vi "Post-Install Custom Action.vi"(10 "Variant":variant) -> (0 "error out":errorcluster)   [LabVIEW 2021]
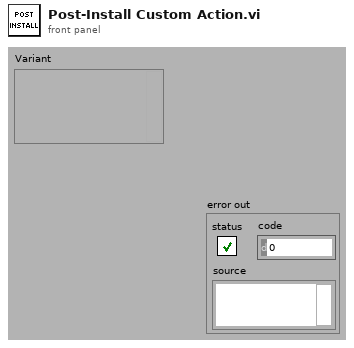
[diagram p1: front panel]
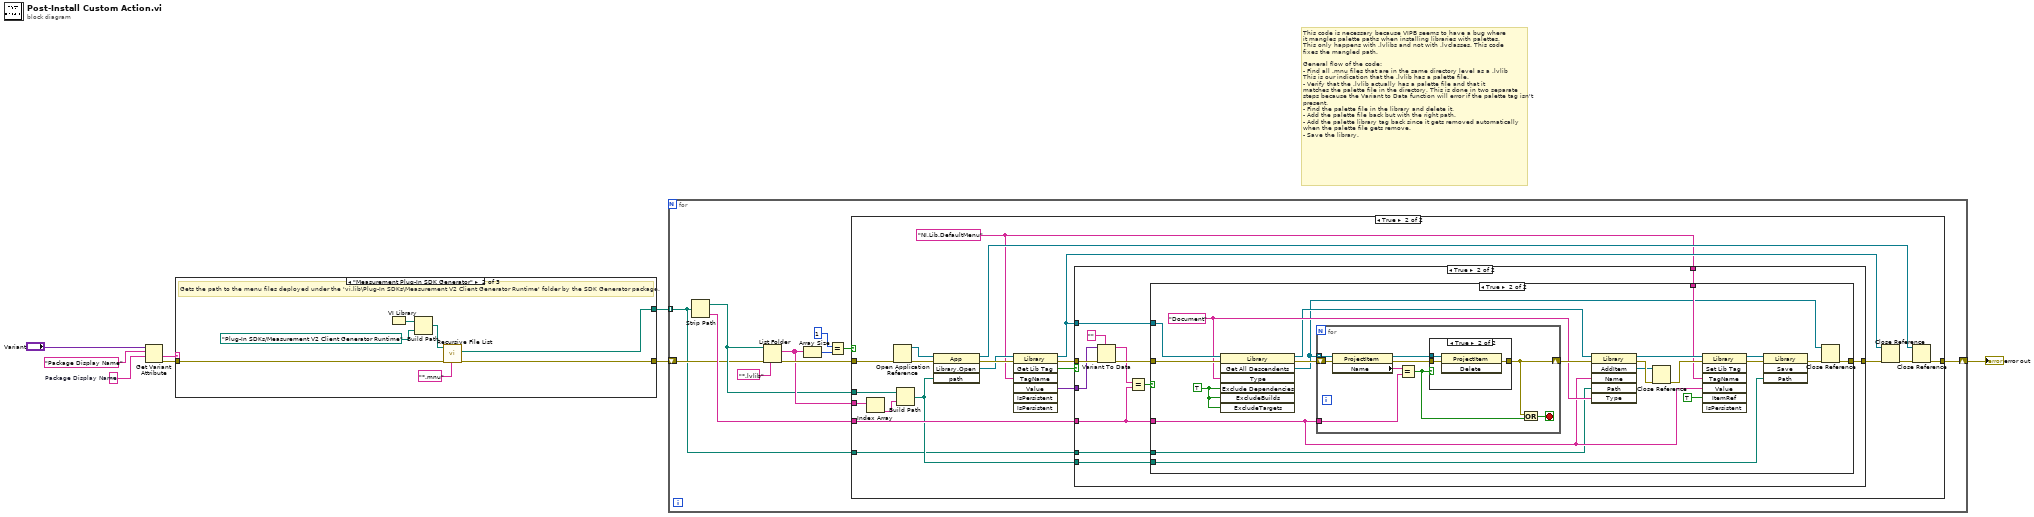
[diagram p0: block diagram]
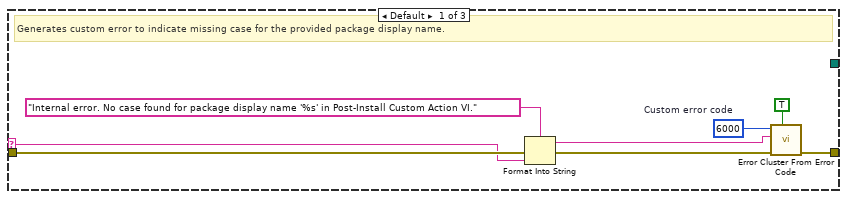
[diagram p6: hidden frame]
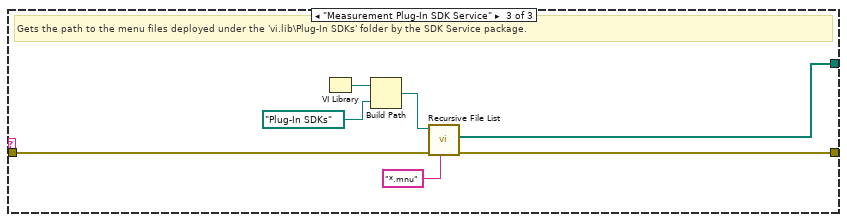
[diagram p7: hidden frame]
diagram:
  w7 = ""  # Package Display Name
  # "This code is necessary because VIPB seems to have a bug where\nit mangles palette paths when installing libraries with palettes.\nThis only happens with .lvlibs and not with .lvclasses. This code\nfixes the mangled path.\n\nGeneral flow of the code:\n- Find all .mnu files that are in the same directory level as a .lvlib\nThis is our indication that the .lvlib has a palette file.\n- Verify that the .lvlib actually has a palette file and that it\nmatches the palette file in the directory. This is done in two separate\nsteps because the Variant to Data function will error if the palette tag isn't\npresent.\n- Find the palette file in the library and delete it.\n- Add the palette file back but with the right path.\n- Add the palette library tag back since it gets removed automatically\nwhen the palette file gets remove.\n- Save the library."
  n1 = Get Variant Attribute(Variant="Variant", name="Package Display Name", default value (empty Variant)=w7) -> (value=w2:string, error out=w1:errorcluster)  [unwired: 1 in, 2 out]
  n2 = case shown="\"Measurement Plug-In SDK Generator\"" w2 {
    selector: w2 -> [w13 _ _]
    tunnel: [_ w18 w27] -> w3
    tunnel: [w16 w19 w28] -> w4
    tunnel: w1 -> [w14 w17 w26]
    frame Default {
      w11 = 6000  # Custom error code
      # "Generates custom error to indicate missing case for the provided package display name."
      n3 = Format Into String(format string="Internal error. No case found for package display name '%s' in Post-Install Custom Action VI.", error in=w14, w13) -> (resulting string=w12:string, error out=w15:errorcluster)  [unwired: 1 in]
      n4 = call <vilib>:"Error Cluster From Error Code.vi"("show call chain? (False)"=TRUE, "error in (no error)"=w15, "error message (\"\")"=w12, "error code (0)"=w11) -> ("error out"=w16:errorcluster)  [unwired: 5 in]
    }
    frame "Measurement Plug-In SDK Generator" {
      # "Gets the path to the menu files deployed under the 'vi.lib\\Plug-In SDKs\\Measurement V2 Client Generator Runtime' folder by the SDK Generator package."
      n5 = VI Library() -> (path=w22:path)
      n6 = Build Path(base path=w22, name or relative path=path "Plug-In SDKs/Measurement V2 Client Generator Runtime") -> (appended path=w23:path)
      n7 = call <vilib>:"Recursive File List.vi"("pattern"="*.mnu", "error in (no error)"=w17, "Folder Path"=w23) -> ("error out"=w19:errorcluster, "All Files in Dir"=w18:path[])  [unwired: 4 in, 3 out]
    }
    frame "Measurement Plug-In SDK Service" {
      # "Gets the path to the menu files deployed under the 'vi.lib\\Plug-In SDKs' folder by the SDK Service package."
      n8 = VI Library() -> (path=w25:path)
      n9 = Build Path(base path=w25, name or relative path=path "Plug-In SDKs") -> (appended path=w30:path)
      n10 = call <vilib>:"Recursive File List.vi"("pattern"="*.mnu", "error in (no error)"=w26, "Folder Path"=w30) -> ("error out"=w28:errorcluster, "All Files in Dir"=w27:path[])  [unwired: 4 in, 3 out]
    }
  }
  n11 = for {
    shift-right: [w33] -> w6
    shift-left: w4 -> [w32]
    tunnel: w3 -> [w31] mode=indexing
    n12 = Strip Path(path=w31) -> (stripped path=w35:path, name=w39:string)
    n13 = List Folder(path=w35, pattern="*.lvlib", error in=w32) -> (filenames=w37:string[], error out=w38:errorcluster)  [unwired: 1 in, 2 out]
    n14 = Array Size(array=w37) -> (size(s)=w41:i32)
    n15 = Equal?(x=1, y=w41) -> (x = y?=w40:bool)
    n16 = case shown="True" w40 {
      tunnel: w38 -> [w42 w59]
      tunnel: w37 -> [_ w62]
      tunnel: w39 -> [_ w54]
      tunnel: w35 -> [_ w50]
      tunnel: [w42 w44] -> w33
      tunnel: w31 -> [_ w43]
      frame False {
      }
      frame True {
        w46 = "NI.Lib.DefaultMenu" ("Tag Name")
        n17 = Index Array(array=w62) -> (element=w49:string)  [unwired: 1 in]
        n18 = Open Application Reference(8:w59) -> (0:w61:errorcluster, 3:w60:refnum<vi>)  [unwired: 3 in]
        n19 = Build Path(base path=w50, name or relative path=w49) -> (appended path=w48:path)
        n20 = invoke class="App" method="Library.Open"(reference=w60, error in=w61, "path"=w48) -> (reference out=w51:refnum<vi>, error out=w58:errorcluster, "Open Library"=w55:refnum<vi>)  [unwired: 1 in, 1 out]
        n21 = invoke class="Library" method="Get Lib Tag"(reference=w55, error in=w58, "TagName"=w46) -> (reference out=w52:refnum<vi>, error out=w56:errorcluster, "GetTag"=w47:bool, "Value"=w57:variant)  [unwired: 4 in, 3 out]
        n22 = case shown="True" w47 {
          tunnel: w57 -> [_ w71]
          tunnel: w56 -> [w63 w72]
          tunnel: [w63 w75] -> w53
          tunnel: w52 -> [_ w74]
          tunnel: w48 -> [_ w73]
          tunnel: w54 -> [_ w67]
          tunnel: w46 -> [_ w65]
          tunnel: w43 -> [_ w64]
          frame False {
          }
          frame True {
            n23 = Variant To Data(error in=w72, type="", Variant=w71) -> (data=w68:string, error out=w70:errorcluster)
            n24 = Equal?(x=w68, y=w67) -> (x = y?=w66:bool)
            n25 = case shown="True" w66 {
              tunnel: [w76 w86] -> w75
              tunnel: w74 -> [_ w97]
              tunnel: w73 -> [_ w92]
              tunnel: w70 -> [w76 w91]
              tunnel: w67 -> [_ w78]
              tunnel: w65 -> [_ w83]
              tunnel: w64 -> [_ w77]
              frame False {
              }
              frame True {
                w85 = "Document" ("Type")
                w81 = TRUE ("ExcludeDependencies")
                n26 = invoke class="Library" method="Get All Descendents"(reference=w97, error in=w91, "Type"=w85, "Exclude Dependencies"=w81, "ExcludeBuilds"=w81, "ExcludeTargets"=w81) -> (reference out=w80:refnum<vi>, error out=w96:errorcluster, "All Descendents"=w79:refnum<vi>[])  [unwired: 1 in, 4 out]
                n27 = for {
                  tunnel: w79 -> [w106] mode=indexing
                  shift-right: [w100] -> w95
                  shift-left: w96 -> [w102]
                  tunnel: w78 -> [w101]
                  stop <- w98 stop-if-true
                  n28 = property class="ProjectItem"(reference=w106, error in=w102) -> (reference out=w104:refnum<vi>, error out=w103:errorcluster, "Name"=w105:string)
                  n29 = Equal?(x=w105, y=w101) -> (x = y?=w99:bool)
                  n30 = case shown="True" w99 {
                    tunnel: w104 -> [_ w110]
                    tunnel: w103 -> [w107 w108]
                    tunnel: [w107 w109] -> w100
                    frame False {
                    }
                    frame True {
                      n31 = invoke class="ProjectItem" method="Delete"(reference=w110, error in=w108) -> (error out=w109:errorcluster)  [unwired: 1 in, 2 out]
                    }
                  }
                  n32 = Or(x=w100, y=w99) -> (x .or. y?=w98:bool)
                }
                n33 = invoke class="Library" method="AddItem"(reference=w80, error in=w95, "Name"=w78, "Path"=w77, "Type"=w85) -> (reference out=w84:refnum<vi>, error out=w89:errorcluster, "AddItem"=w88:refnum<vi>)  [unwired: 1 in, 3 out]
                n34 = Close Reference(reference=w88, error in (no error)=w89) -> (error out=w87:errorcluster)
                n35 = invoke class="Library" method="Set Lib Tag"(reference=w84, error in=w87, "TagName"=w83, "Value"=w78, "ItemRef"=TRUE ("Is Persistent")) -> (reference out=w94:refnum<vi>, error out=w93:errorcluster)  [unwired: 2 in, 5 out]
                n36 = invoke class="Library" method="Save"(reference=w94, error in=w93, "Path"=w92) -> (error out=w90:errorcluster)  [unwired: 1 in, 3 out]
                n37 = Close Reference(reference=w79, error in (no error)=w90) -> (error out=w86:errorcluster)
              }
            }
          }
        }
        n38 = Close Reference(reference=w52, error in (no error)=w53) -> (error out=w45:errorcluster)
        n39 = Close Reference(reference=w51, error in (no error)=w45) -> (error out=w44:errorcluster)
      }
    }
  }
  "error out" <- w6
